vi "CSV File to fWform.vi"(1 "CSV Path IN":path, 5 "error in (no error)":errorcluster) -> (11 "CSV Path OUT":path, 13 "wForms":waveform(dbl)[](array[waveform]), 19 "error out":errorcluster)   [LabVIEW 2022 SP3, in "TEXT.lvclass"]
uses:
  TEXT.lvclass
panel:
  out "Nb Samples":i32
  out "Nb Signals":i32
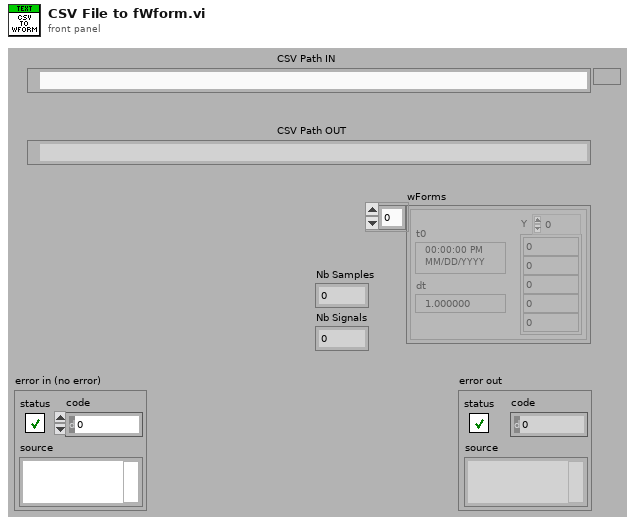
[diagram p1: front panel]
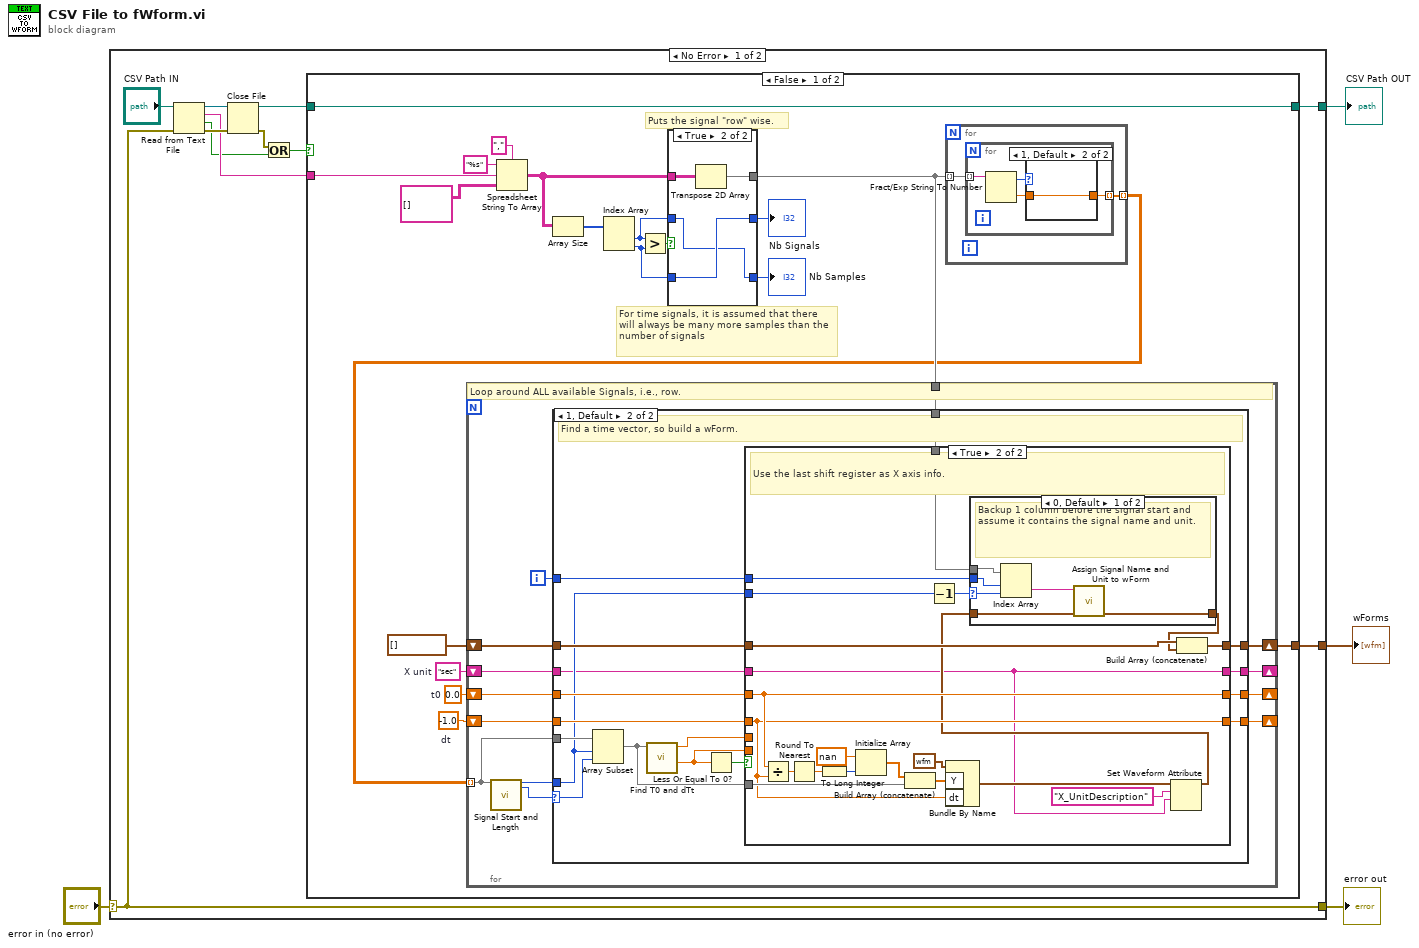
[diagram p0: block diagram]
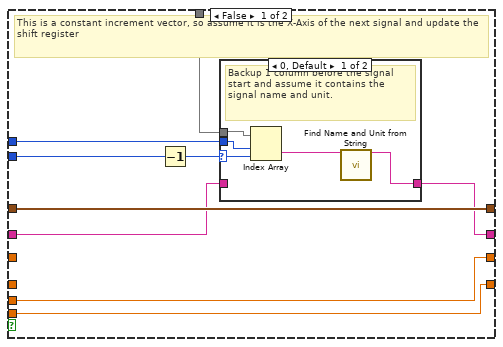
[diagram p3: hidden frame]
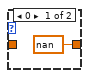
[diagram p6: hidden frame]
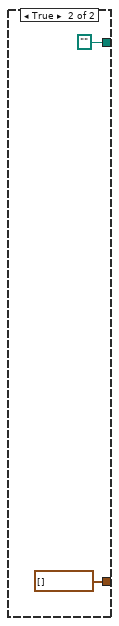
[diagram p8: hidden frame]
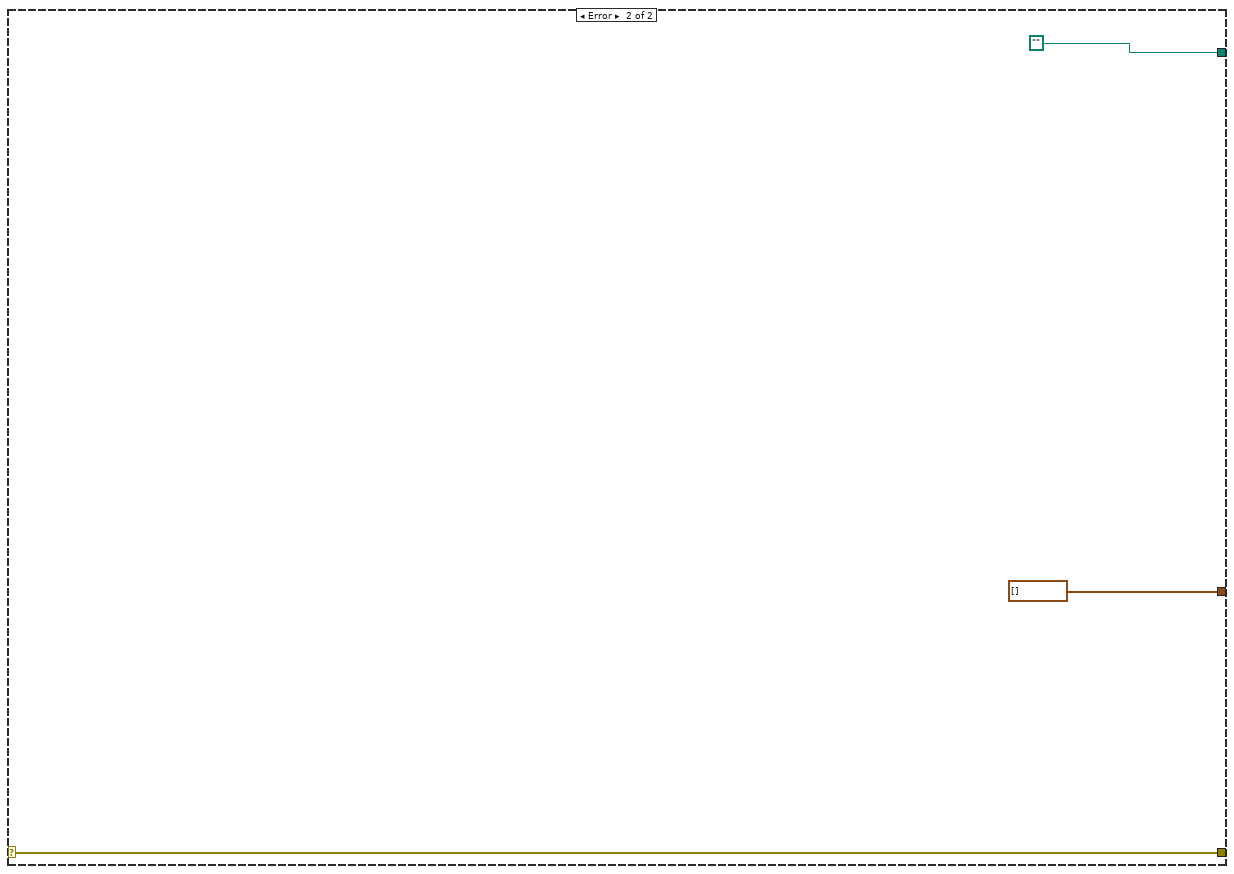
[diagram p9: hidden frame]
diagram:
  n1 = case shown="No Error" "error in (no error)" {
    selector: "error in (no error)" -> [w11 w131]
    tunnel: [w11 w131] -> w3
    tunnel: [w6 path ""] -> w2
    tunnel: [w15 waveform(dbl)[] [] ("wForms")] -> w1
    frame No Error {
      n2 = Read from Text File(file (use dialog)="CSV Path IN", error in=w11) -> (refnum out=w12:refnum<file>, text=w10:string, cancelled=w8:bool, error out=w13:errorcluster)  [unwired: 2 in]
      n3 = Close File(refnum=w12, error in=w13) -> (path=w5:path, error out=w9:errorcluster)
      n4 = Or(x=w9, y=w8) -> (x .or. y?=w7:bool)
      n5 = case shown="False" w7 {
        tunnel: [w23 waveform(dbl)[] []] -> w15
        tunnel: w10 -> [w20 _]
        tunnel: [w17 path ""] -> w6
        tunnel: w5 -> [w17 _]
        frame False {
          w16 = "sec"  # X unit
          w31 = -1.0  # dt
          w30 = 0.0  # t0
          # "Puts the signal \"row\" wise."
          # "For time signals, it is assumed that there will always be many more samples than the number of signals"
          n6 = Spreadsheet String To Array(delimiter (Tab)=",", format string="%s", spreadsheet string=w20, array type (2D Dbl)=string[][] []) -> (array=w18:string[][])
          n7 = Array Size(array=w18) -> (size(s)=w24:i32[])
          n8 = Index Array(array=w24) -> (element #1=w27:i32, element #2=w29:i32)  [unwired: 2 in]
          n9 = Greater?(x=w27, y=w29) -> (0:w25:bool)
          n10 = case shown="True" w25 {
            tunnel: w18 -> [w122 w126]
            tunnel: [w122 w125] -> w34
            tunnel: [w121 w124] -> w26
            tunnel: w27 -> [w121 w123]
            tunnel: [w120 w123] -> w28
            tunnel: w29 -> [w120 w124]
            frame False {
            }
            frame True {
              n11 = Transpose 2D Array(2D array=w126) -> (transposed array=w125:string[][])
            }
          }
          "Nb Samples" <- w28
          "Nb Signals" <- w26
          n12 = for {
            tunnel: w34 -> [w113] mode=indexing
            tunnel: [w112] -> w33 mode=indexing
            n13 = for {
              tunnel: w113 -> [w117] mode=indexing
              tunnel: [w115] -> w112 mode=indexing
              n14 = Fract/Exp String To Number(string=w117) -> (offset past number=w116:i32, number=w114:dbl)  [unwired: 3 in]
              n15 = case shown="1, Default" w116 {
                tunnel: [nan w119] -> w115
                tunnel: w114 -> [_ w119]
                frame 0 {
                }
                frame 1, Default {
                }
              }
            }
          }
          n16 = for {
            shift-right: [w42] -> w23
            shift-left: waveform(dbl)[] [] -> [w41]
            tunnel: w33 -> [w45] mode=indexing
            shift-right: [w44] -> _
            shift-left: w30 -> [w40]
            shift-right: [w43] -> _
            shift-left: w31 -> [w39]
            tunnel: w34 -> [w37]
            shift-right: [w36] -> _
            shift-left: w16 -> [w35]
            i -> [w38]
            # "Loop around ALL available Signals, i.e., row."
            n17 = call "Signal Start and Length.vi"("Time Signal IN"=w45) -> ("Start Index"=w46:i32, "Length"=w47:i32)  [unwired: 17 in]
            n18 = case shown="1, Default" w47 {
              selector: w47 -> [_ w68]
              tunnel: w46 -> [_ w59]
              tunnel: w45 -> [_ w67]
              tunnel: [w50 w65] -> w44
              tunnel: [w49 w64] -> w43
              tunnel: [w51 w63] -> w42
              tunnel: w41 -> [w51 w62]
              tunnel: w40 -> [w50 w61]
              tunnel: w39 -> [w49 w60]
              tunnel: w38 -> [_ w58]
              tunnel: w37 -> [_ w57]
              tunnel: [w48 w53] -> w36
              tunnel: w35 -> [w48 w52]
              frame 0 {
                # "No time vector found, so do nothing and continue to the next \"vector\""
              }
              frame 1, Default {
                # "Find a time vector, so build a wForm."
                n19 = Array Subset(array=w67, index=w59, length=w68) -> (w56:dbl[])
                n20 = call "Find T0 and dTt.vi"("Array"=w56) -> ("dT"=w55:dbl, "T0"=w54:dbl)  [unwired: 9 in]
                n21 = Less Or Equal To 0?(x=w55) -> (x <= 0?=w66:bool)
                n22 = case shown="True" w66 {
                  tunnel: [w77 w94] -> w65
                  tunnel: w54 -> [w77 _]
                  tunnel: [w76 w93] -> w64
                  tunnel: w55 -> [w76 _]
                  tunnel: w56 -> [_ w98]
                  tunnel: [w75 w96] -> w63
                  tunnel: w62 -> [w75 w95]
                  tunnel: w61 -> [_ w94]
                  tunnel: w60 -> [_ w93]
                  tunnel: w59 -> [w72 w92]
                  tunnel: w58 -> [w73 w90]
                  tunnel: w57 -> [w74 w89]
                  tunnel: [w70 w84] -> w53
                  tunnel: w52 -> [w69 w84]
                  frame False {
                    # "This is a constant increment vector, so assume it is the X-Axis of the next signal and update the shift register"
                    n23 = Decrement(x=w72) -> (x-1=w71:i32)
                    n24 = case shown="0, Default" w71 {
                      selector: w71 -> [w80 _]
                      tunnel: w73 -> [w82 _]
                      tunnel: w74 -> [w81 _]
                      tunnel: [w78 w83] -> w70
                      tunnel: w69 -> [_ w83]
                      frame 0, Default {
                        # "Backup 1 column before the signal start and assume it contains the signal name and unit."
                        n25 = Index Array(array=w81, index (row)=w82, index (col)=w80) -> (element=w79:string)
                        n26 = call "Find Name and Unit from String.vi"("Input String"=w79) -> ("Units"=w78:string)  [unwired: 17 in, 1 out]
                      }
                      frame ..-1 {
                        # "The signal starts at the very first column, so there are NO header column/info"
                      }
                    }
                  }
                  frame True {
                    # "Use the last shift register as X axis info."
                    n27 = Divide(x=w94, y=w93) -> (x/y=w103:dbl)
                    n28 = Round To Nearest(number=w103) -> (nearest integer value=w102:dbl)
                    n29 = To Long Integer(number=w102) -> (32bit integer=w101:i32)
                    n30 = Initialize Array(nan ("element"), w101) -> (w99:dbl[])
                    n31 = Build Array (concatenate)(w99, w98) -> (w97:dbl[])
                    n32 = Decrement(x=w92) -> (x-1=w91:i32)
                    n33 = Bundle By Name(cluster=waveform(dbl) {"t0"=timestamp(0 s since 1904-01-01), "dt"=1.0, "Y"=[]} ("Waveform"), "Y"=w97, "dt"=w93) -> (w86:waveform(dbl))
                    n34 = Set Waveform Attribute(5:w84, 6:"X_UnitDescription" ("Att - X unit"), 7:w86) -> (3:w85:waveform(dbl))  [unwired: 1 in, 2 out]
                    n35 = case shown="0, Default" w91 {
                      selector: w91 -> [w108 _]
                      tunnel: [w105 w111] -> w88
                      tunnel: w85 -> [w106 w111]
                      tunnel: w90 -> [w110 _]
                      tunnel: w89 -> [w109 _]
                      frame 0, Default {
                        # "Backup 1 column before the signal start and assume it contains the signal name and unit."
                        n36 = Index Array(array=w109, index (row)=w110, index (col)=w108) -> (element=w107:string)
                        n37 = call "Assign Signal Name and Unit to wForm.vi"("wform IN"=w106, "Input String"=w107) -> ("wform OUT"=w105:waveform(dbl))  [unwired: 9 in]
                      }
                      frame ..-1 {
                        # "The signal starts at the very first column, so there are NO header column/info"
                      }
                    }
                    n38 = Build Array (concatenate)(w95, w88) -> (w96:waveform(dbl)[])
                  }
                }
              }
            }
          }
        }
        frame True {
        }
      }
    }
    frame Error {
    }
  }
  "error out" <- w3
  "CSV Path OUT" <- w2
  "wForms" <- w1
